vi "Simple Actor Show.vi"   [LabVIEW 2020, in "Simple Actor.lvlib"]
uses:
  Simple Actor.lvlib
  Simple Actor/Simple Actor.lvclass
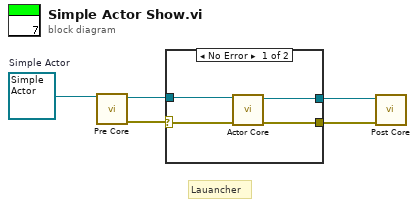
[diagram p0: block diagram]
diagram:
  w5 = refnum<class "Simple Actor.lvclass"> refnum  # Simple Actor
  # "Lauancher"
  n1 = call-dynamic "Pre Core.vi"("Simple Actor in"=w5) -> ("error out"=w4:errorcluster, "Simple Actor out"=w3:refnum<class "Simple Actor.lvclass">)  [unwired: 9 in]
  n2 = case shown="No Error" w4 {
    selector: w4 -> [w9 w10]
    tunnel: w3 -> [w8 w11]
    tunnel: [w7 w11] -> w2
    tunnel: [w6 w10] -> w1
    frame No Error {
      n3 = call-dynamic "Actor Core.vi"("error in (no error)"=w9, "Simple Actor in"=w8) -> ("error out"=w6:errorcluster, "Simple Actor out"=w7:refnum<class "Simple Actor.lvclass">)  [unwired: 8 in]
    }
    frame Error {
    }
  }
  n4 = call-dynamic "Post Core.vi"("error in (no error)"=w1, "Simple Actor in"=w2) -> ()  [unwired: 8 in, 2 out]
